vi "imaging gate sweep v1.1.vi"() -> ()   [LabVIEW 2021]
uses:
  <userlib>/Nanonis Prog Interface V5/Nanonis Prog Interface.lvlib
panel:
  in  "Time/Frame (s)":dbl
  in  "Tip move speed (m/s)":dbl=1e-09 format="%#_6p"
  in  "Home\nafter?":bool
  in  "milliseconds to wait":u32
  in  "Direction: \nUp\n\n\nDown":bool=TRUE
  in  "Serie name":string caption="Basename (empty= no change)"
  in  "Gate increment (V)":dbl
  in  "End gate (V)":dbl
  in  "Start gate (V)":dbl
  # "KPN: Correct Imaging vs. Gate voltage program, 8/9/22"
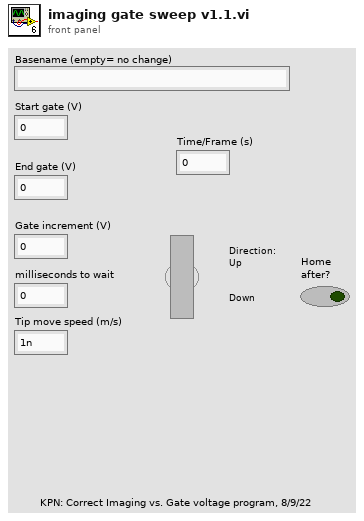
[diagram p1: front panel]
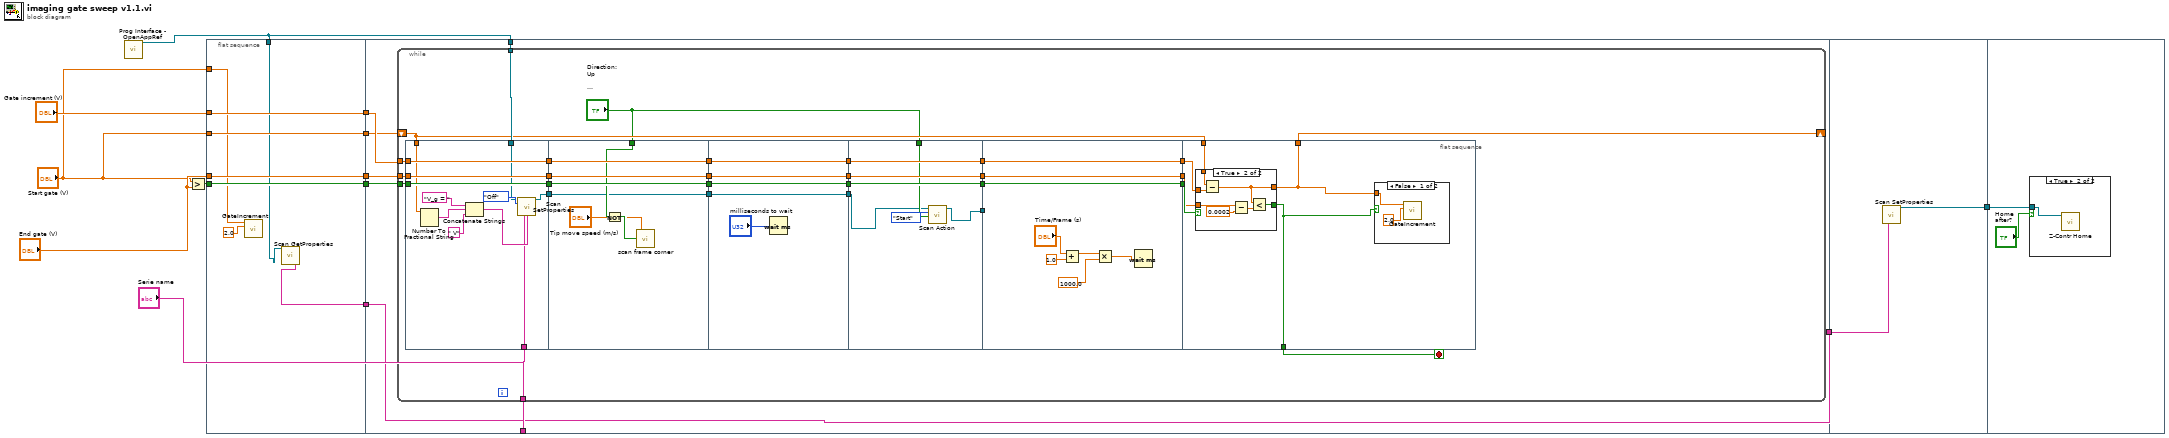
[diagram p0: block diagram]
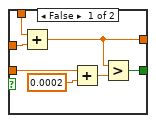
[diagram p3: hidden frame]
diagram:
  n1 = call <userlib>:"Prog Interface - OpenAppRef.vi"() -> ("Application reference"=w2:refnum<vi>)  [unwired: 6 in, 1 out]
  n2 = Greater?(x="Start gate (V)", y="End gate (V)") -> (0:w13:bool)
  n3 = flat-sequence {
    tunnel: "End gate (V)" -> [w18]
    tunnel: "Start gate (V)" -> [w19]
    tunnel: "Gate increment (V)" -> [w20]
    tunnel: w13 -> [w21]
    tunnel: [w21] -> w10
    tunnel: [w20] -> w9
    tunnel: [w19] -> w8
    tunnel: [w18] -> w7
    tunnel: "Start gate (V)" -> [w16]
    tunnel: [w15] -> w4
    tunnel: w2 -> [w14]
    tunnel: w10 -> [w28]
    tunnel: w9 -> [w27]
    tunnel: w8 -> [w26]
    tunnel: w7 -> [w25]
    tunnel: w2 -> [w24]
    tunnel: "Serie name" -> [w23]
    tunnel: w4 -> [w22]
    tunnel: [w22] -> w3
    tunnel: w3 -> [w119]
    tunnel: [w118] -> w1
    tunnel: w1 -> [w121]
    frame #0 {
      n4 = call "GateIncrement.vi"("Increment"=2.0, "Gate Voltage"=w16) -> ()  [unwired: 10 in]
      n5 = call <userlib>:"Scan GetProperties.vi"("Application ref in"=w14) -> ("Serie name"=w15:string)  [unwired: 7 in, 7 out]
    }
    frame #1 {
      n6 = while {
        tunnel: w28 -> [w56]
        tunnel: w27 -> [w55]
        shift-right: [w47] -> _
        shift-left: w26 -> [w48]
        tunnel: w25 -> [w54]
        tunnel: w24 -> [w50]
        tunnel: w23 -> [w49]
        stop <- w29 stop-if-true
        n7 = flat-sequence {
          tunnel: w54 -> [w66]
          tunnel: w55 -> [w67]
          tunnel: w56 -> [w68]
          tunnel: [w68] -> w46
          tunnel: [w67] -> w44
          tunnel: [w66] -> w42
          tunnel: w48 -> [w62]
          tunnel: w50 -> [w59]
          tunnel: [w58] -> w40
          tunnel: w49 -> [w57]
          tunnel: w46 -> [w75]
          tunnel: [w75] -> w45
          tunnel: w44 -> [w74]
          tunnel: [w74] -> w43
          tunnel: w42 -> [w73]
          tunnel: [w73] -> w41
          tunnel: w40 -> [w69]
          tunnel: "Direction: \nUp\n\n\nDown" -> [w72]
          tunnel: [w69] -> w30
          tunnel: [w80] -> w38
          tunnel: [w79] -> w37
          tunnel: [w78] -> w36
          tunnel: [w77] -> w31
          tunnel: w30 -> [w77]
          tunnel: w45 -> [w80]
          tunnel: w43 -> [w79]
          tunnel: w41 -> [w78]
          tunnel: w38 -> [w87]
          tunnel: [w87] -> w35
          tunnel: w37 -> [w86]
          tunnel: [w86] -> w34
          tunnel: w36 -> [w85]
          tunnel: [w85] -> w33
          tunnel: [w84] -> w32
          tunnel: "Direction: \nUp\n\n\nDown" -> [w83]
          tunnel: w31 -> [w81]
          tunnel: [w95] -> w53
          tunnel: [w94] -> w52
          tunnel: [w93] -> w51
          tunnel: w32 -> [_]
          tunnel: w33 -> [w93]
          tunnel: w34 -> [w94]
          tunnel: w35 -> [w95]
          tunnel: w51 -> [w99]
          tunnel: w52 -> [w100]
          tunnel: w53 -> [w101]
          tunnel: [w98] -> w29
          tunnel: w48 -> [w97]
          tunnel: [w96] -> w47
          frame #0 {
            n8 = Number To Fractional String(number=w62) -> (F-format string=w65:string)  [unwired: 3 in]
            n9 = Concatenate Strings("V_g = " ("string"), w65, " V" ("string")) -> (w61:string)
            n10 = call <userlib>:"Scan SetProperties.vi"("Application ref in"=w59, "Continuous scan"=enum16{"No change", "On", "Off"}."Off", "Serie name"=w57, "Comment"=w61) -> ("Application ref out"=w58:refnum<vi>)  [unwired: 10 in, 1 out]
          }
          frame #1 {
            n11 = Not(x=w72) -> (.not. x?=w71:bool)
            n12 = call "scan frame corner.vi"("Speed (m/s)"="Tip move speed (m/s)", "Corner (T = top left, F = bottom left)"=w71) -> ()
          }
          frame #2 {
            n13 = Wait (ms)(milliseconds to wait="milliseconds to wait") -> ()  [unwired: 1 out]
          }
          frame #3 {
            n14 = call <userlib>:"Scan Action.vi"("Direction: up/down (T=up)"=w83, "Scan action (Start)"=enum16{"Start", "Stop", "Pause", "Resume"}."Start", "Application ref in"=w81) -> ("Application ref out"=w84:refnum<vi>)  [unwired: 6 in, 1 out]
          }
          frame #4 {
            n15 = Add(x="Time/Frame (s)", y=1.0) -> (x+y=w90:dbl)
            n16 = Multiply(x=w90, y=1000.0) -> (x*y=w88:dbl)
            n17 = Wait (ms)(milliseconds to wait=w88) -> ()  [unwired: 1 out]
          }
          frame #5 {
            n18 = case shown="True" w101 {
              tunnel: w100 -> [w110 w117]
              tunnel: [w105 w115] -> w96
              tunnel: w99 -> [w109 w114]
              tunnel: [w107 w116] -> w98
              tunnel: w97 -> [w104 w111]
              frame False {
                n19 = Add(x=w104, y=w110) -> (x+y=w105:dbl)
                n20 = Add(x=w109, y=0.0002) -> (x+y=w106:dbl)
                n21 = Greater?(x=w105, y=w106) -> (0:w107:bool)
              }
              frame True {
                n22 = Subtract(x=w111, y=w117) -> (x-y=w115:dbl)
                n23 = Subtract(x=w114, y=0.0002) -> (x-y=w112:dbl)
                n24 = Less?(x=w115, y=w112) -> (x < y?=w116:bool)
              }
            }
            n25 = case shown="False" w98 {
              tunnel: w96 -> [w103 _]
              frame False {
                n26 = call "GateIncrement.vi"("Increment"=2.0, "Gate Voltage"=w103) -> ()  [unwired: 10 in]
              }
              frame True {
              }
            }
          }
        }
      }
    }
    frame #2 {
      n27 = call <userlib>:"Scan SetProperties.vi"("Serie name"=w119) -> ("Application ref out"=w118:refnum<vi>)  [unwired: 13 in, 1 out]
    }
    frame #3 {
      n28 = case shown="True" "Home\nafter?" {
        tunnel: w121 -> [_ w122]
        frame False {
        }
        frame True {
          n29 = call <userlib>:"Z-Contr Home.vi"("Application ref in"=w122) -> ()  [unwired: 9 in, 2 out]
        }
      }
    }
  }
